vi "Close Session.vi"(0 "session in":refnum<k21>, 11 "error in (no error)":errorcluster) -> (15 "error out":errorcluster)   [LabVIEW 2020, in "SLSC.lvlib"]
doc: "Closes an SLSC session."
uses:
  <vilib>/SLSC/SLSC.lvlib
  nislsclvapi.dll
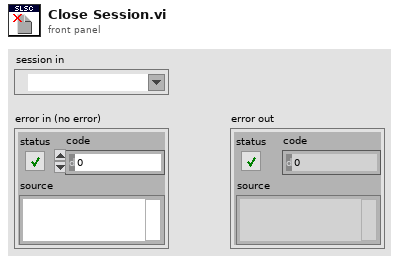
[diagram p1: front panel]
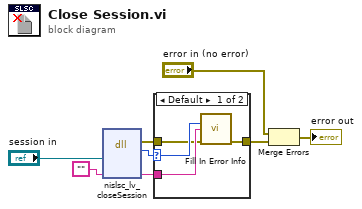
[diagram p0: block diagram]
diagram:
  n1 = dll-call lib="nislsclvapi.*" fn="nislsc_lv_closeSession"("session"="session in", "extendedErrorInfo"="") -> (error out=w2:errorcluster, "return type"=w3:i32, "extendedErrorInfo"=w4:string)  [unwired: 6 in, 1 out]
  n2 = case shown="Default" w3 {
    selector: w3 -> [w12 _]
    tunnel: w4 -> [w11 _]
    tunnel: w2 -> [w10 w13]
    tunnel: [w9 w13] -> w1
    frame Default {
      n3 = call <vilib>:"Fill In Error Info.vi"("status code"=w12, "extended error info"=w11, "error in"=w10) -> ("error out"=w9:errorcluster)  [unwired: 12 in]
    }
    frame 0 {
    }
  }
  n4 = Merge Errors("error in (no error)", w1) -> (→"error out":errorcluster)
